vi "adjustAngle_03.vi"() -> ()   [LabVIEW 2011]
panel:
  out "dtArray":dbl[](array[numeric])
  out "t0":dbl
  in  "points to watch":i32
  in  "first":bool=TRUE
  in  "tArray":dbl[](array[numeric])
  out "tStart":dbl
  out "Measure":bool
  in  "Move to ref angle first":bool=TRUE
  in  "time done (s)":dbl
  in  "time to wait (s)":dbl=2.0
  out "Wait to set":bool
  in  "Ref Angle (deg)":dbl=30.0 format="%.1f"
  out "IO error":errorcluster
  in  "stop":bool
  out "Angle Indicator (deg)":dbl=20.6 caption="Angle (deg)" format="%.1f"
  in  "Angle (deg)":dbl format="%.1f"
  out "P (torr)":dbl=19.959999999999997 format="%.2f"
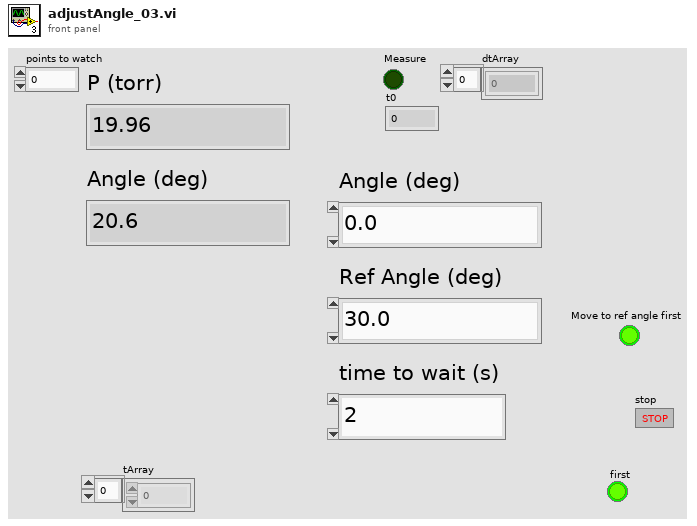
[diagram p1: front panel]
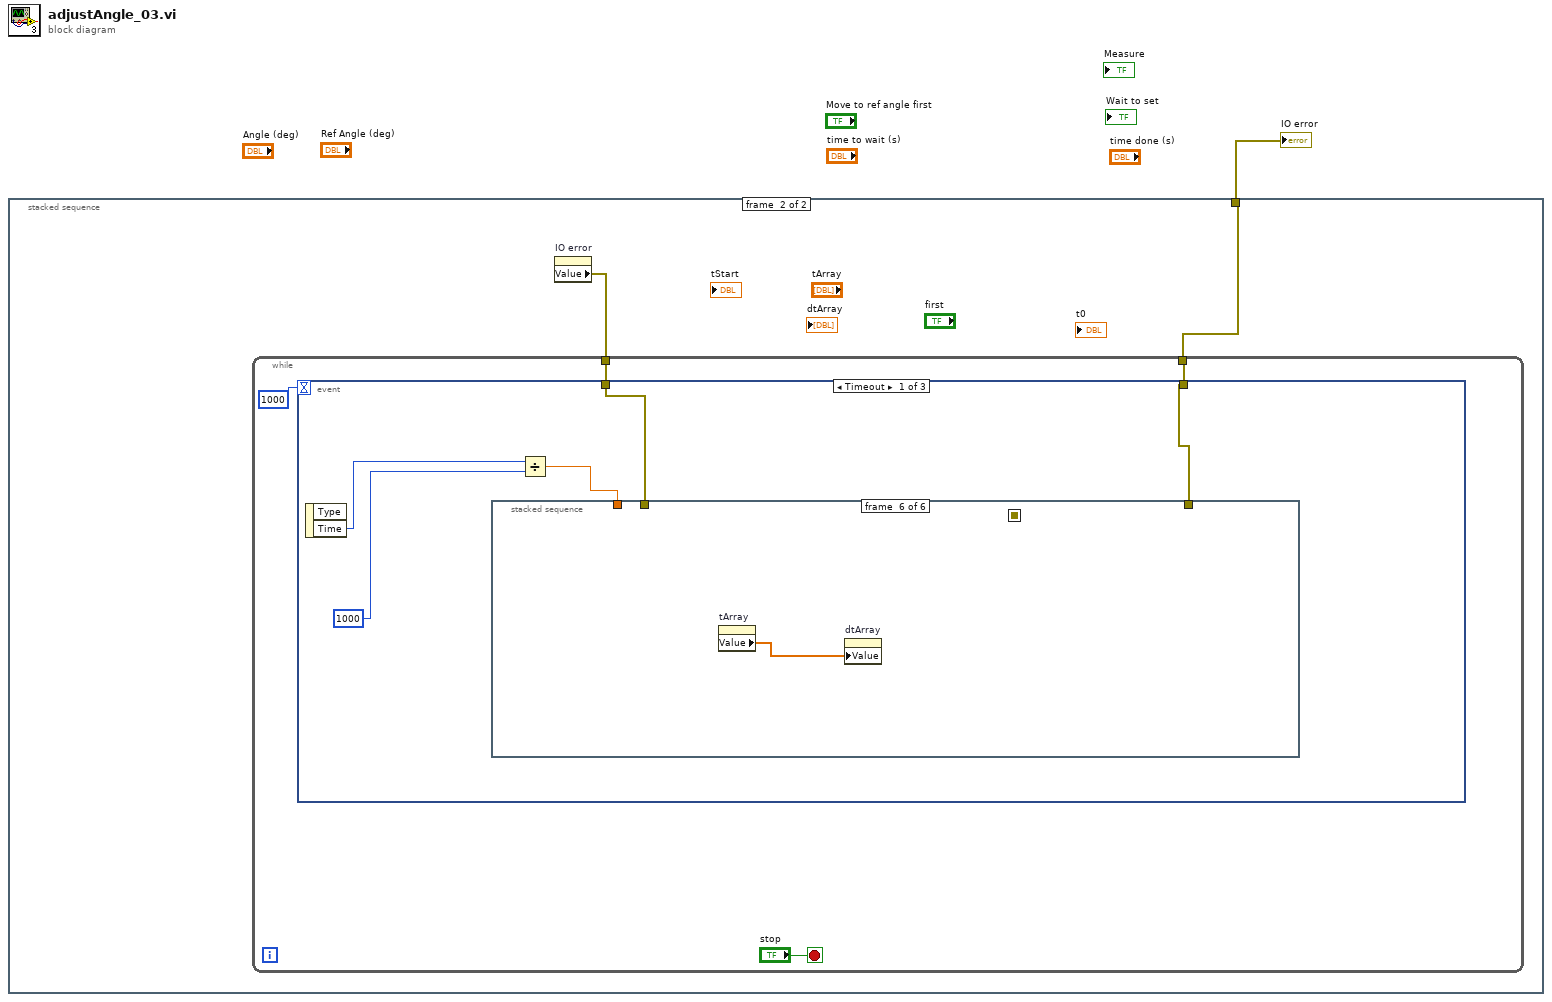
[diagram p0: block diagram]
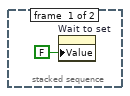
[diagram p2: hidden frame]
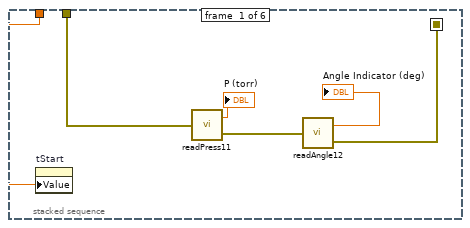
[diagram p3: hidden frame]
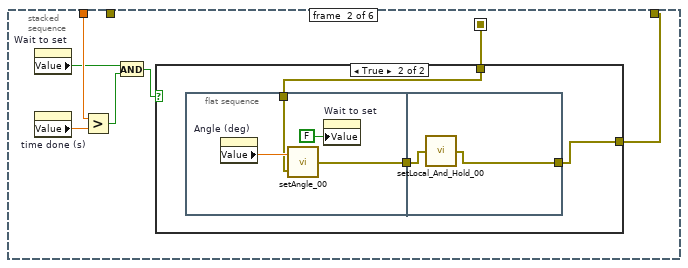
[diagram p4: hidden frame]
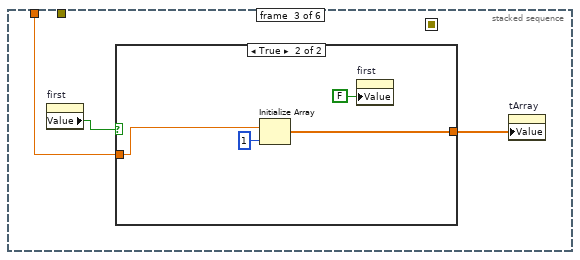
[diagram p6: hidden frame]
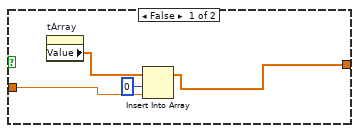
[diagram p7: hidden frame]
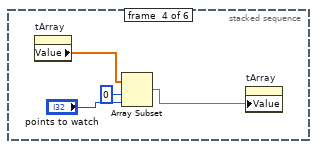
[diagram p8: hidden frame]
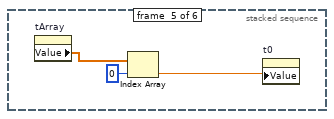
[diagram p9: hidden frame]
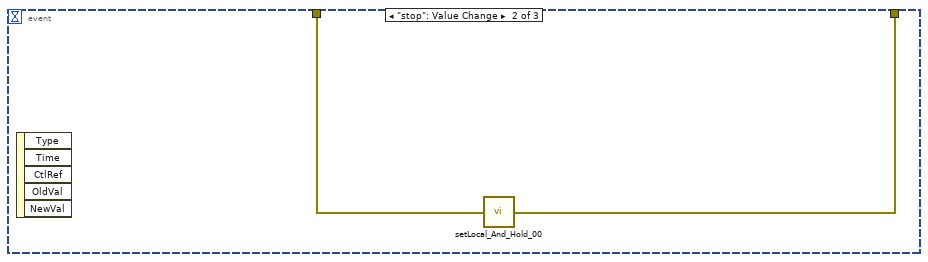
[diagram p10: hidden frame]
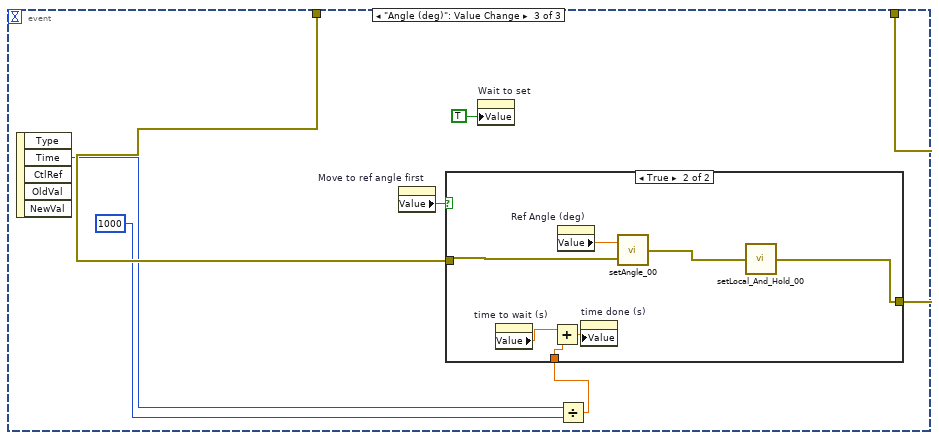
[diagram p11: hidden frame]
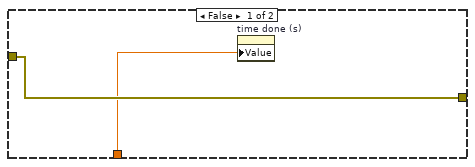
[diagram p12: hidden frame]
diagram:
  n1 = stacked-sequence {
    tunnel: [_ w3] -> w1
    frame #0 {
      n2 = property on="Wait to set" class="Bool (strict)"("Value"=FALSE ("Wait to set")) -> ()  [unwired: 2 in, 2 out]
    }
    frame #1 {
      n3 = property on="IO error" class="Clust (strict)"() -> ("Value"=w4:errorcluster)  [unwired: 2 in, 2 out]
      n4 = while {
        tunnel: w4 -> [w7]
        tunnel: [w6] -> w3
        stop <- "stop" stop-if-true
        n5 = event shown="[0] Timeout" {
          selector: _ -> [_ _ _]
          dyn-events: _ -> [_ _ _]
          timeout: 1000 -> [_ _ _]
          tunnel: w7 -> [w13 w57 w63]
          tunnel: [w12 w56 w64] -> w6
          event Timeout {
            n6 = event-data() -> ("Time"=w11:u32)  [unwired: 1 in, 1 out]
            n7 = Divide(x=w11, y=u32 1000) -> (x/y=w9:dbl)
            n8 = stacked-sequence {
              seq-local: [w15 _ _ _ _ _] -> [_ w20 _ _ _ _]
              tunnel: w13 -> [w19 _ _ _ _ _]
              tunnel: w9 -> [w14 w26 w39 _ _ _]
              tunnel: [_ w22 _ _ _ _] -> w12
              frame #0 {
                n9 = property on="tStart" class="DigNum (strict)"("Value"=w14) -> ()  [unwired: 2 in, 2 out]
                n10 = call "readPress11.vi"("error in"=w19) -> ("P"=→"P (torr)":dbl, "error out"=w16:errorcluster)
                n11 = call "readAngle12.vi"("error in"=w16) -> ("angle"=→"Angle Indicator (deg)":dbl, "error out"=w15:errorcluster)
              }
              frame #1 {
                n12 = property on="Wait to set" class="Bool (strict)"() -> ("Value"=w21:bool)  [unwired: 2 in, 2 out]
                n13 = property on="time done (s)" class="DigNum (strict)"() -> ("Value"=w25:dbl)  [unwired: 2 in, 2 out]
                n14 = Greater?(x=w26, y=w25) -> (0:w24:bool)
                n15 = And(x=w21, y=w24) -> (x .and. y?=w23:bool)
                n16 = case shown="True" w23 {
                  tunnel: [w27 w30] -> w22
                  tunnel: w20 -> [w27 w28]
                  frame False {
                  }
                  frame True {
                    n17 = flat-sequence {
                      tunnel: [w33] -> w29
                      tunnel: w28 -> [w31]
                      tunnel: [w35] -> w30
                      tunnel: w29 -> [w36]
                      frame #0 {
                        n18 = property on="Angle (deg)" class="DigNum (strict)"() -> ("Value"=w34:dbl)  [unwired: 2 in, 2 out]
                        n19 = call "setAngle_00.vi"("error in (no error)"=w31, "Angle (deg)"=w34) -> ("error out"=w33:errorcluster)
                        n20 = property on="Wait to set" class="Bool (strict)"("Value"=FALSE ("Wait to set")) -> ()  [unwired: 2 in, 2 out]
                      }
                      frame #1 {
                        n21 = call "setLocal_And_Hold_00.vi"("error in (no error)"=w36) -> ("error out"=w35:errorcluster)
                      }
                    }
                  }
                }
              }
              frame #2 {
                n22 = property on="first" class="Bool (strict)"() -> ("Value"=w38:bool)  [unwired: 2 in, 2 out]
                n23 = case shown="True" w38 {
                  tunnel: w39 -> [w43 w47]
                  tunnel: [w40 w45] -> w37
                  frame False {
                    n24 = property on="tArray" class="Arr (strict)"() -> ("Value"=w42:dbl[])  [unwired: 2 in, 2 out]
                    n25 = Insert Into Array(array=w42, index=0, new element=w43) -> (w40:dbl[])
                  }
                  frame True {
                    n26 = Initialize Array(w47, 1 ("dimension size")) -> (w45:dbl[])
                    n27 = property on="first" class="Bool (strict)"("Value"=FALSE ("first")) -> ()  [unwired: 2 in, 2 out]
                  }
                }
                n28 = property on="tArray" class="Arr (strict)"("Value"=w37) -> ()  [unwired: 2 in, 2 out]
              }
              frame #3 {
                n29 = property on="tArray" class="Arr (strict)"() -> ("Value"=w49:dbl[])  [unwired: 2 in, 2 out]
                n30 = Array Subset(array=w49, index=0, length="points to watch") -> (w48:dbl[])
                n31 = property on="tArray" class="Arr (strict)"("Value"=w48) -> ()  [unwired: 2 in, 2 out]
              }
              frame #4 {
                n32 = property on="tArray" class="Arr (strict)"() -> ("Value"=w54:dbl[])  [unwired: 2 in, 2 out]
                n33 = Index Array(array=w54, index=0) -> (element=w52:dbl)
                n34 = property on="t0" class="DigNum (strict)"("Value"=w52) -> ()  [unwired: 2 in, 2 out]
              }
              frame #5 {
                n35 = property on="tArray" class="Arr (strict)"() -> ("Value"=w55:dbl[])  [unwired: 2 in, 2 out]
                n36 = property on="dtArray" class="Arr (strict)"("Value"=w55) -> ()  [unwired: 2 in, 2 out]
              }
            }
          }
          event "stop": Value Change {
            n37 = event-data() -> ()  [unwired: 1 in, 5 out]
            n38 = call "setLocal_And_Hold_00.vi"("error in (no error)"=w57) -> ("error out"=w56:errorcluster)
          }
          event "Angle (deg)": Value Change {
            n39 = event-data() -> ("Time"=w62:u32)  [unwired: 1 in, 4 out]
            n40 = property on="Move to ref angle first" class="Bool (strict)"() -> ("Value"=w59:bool)  [unwired: 2 in, 2 out]
            n41 = property on="Wait to set" class="Bool (strict)"("Value"=TRUE ("Wait to set")) -> ()  [unwired: 2 in, 2 out]
            n42 = Divide(x=w62, y=u32 1000) -> (x/y=w60:dbl)
            n43 = case shown="True" w59 {
              tunnel: w63 -> [w66 w72]
              tunnel: [w66 w67] -> w64
              tunnel: w60 -> [w65 w69]
              frame False {
                n44 = property on="time done (s)" class="DigNum (strict)"("Value"=w65) -> ()  [unwired: 2 in, 2 out]
              }
              frame True {
                n45 = property on="time to wait (s)" class="DigNum (strict)"() -> ("Value"=w70:dbl)  [unwired: 2 in, 2 out]
                n46 = Add(x=w70, y=w69) -> (x+y=w71:dbl)
                n47 = property on="Ref Angle (deg)" class="DigNum (strict)"() -> ("Value"=w73:dbl)  [unwired: 2 in, 2 out]
                n48 = property on="time done (s)" class="DigNum (strict)"("Value"=w71) -> ()  [unwired: 2 in, 2 out]
                n49 = call "setAngle_00.vi"("error in (no error)"=w72, "Angle (deg)"=w73) -> ("error out"=w68:errorcluster)
                n50 = call "setLocal_And_Hold_00.vi"("error in (no error)"=w68) -> ("error out"=w67:errorcluster)
              }
            }
          }
        }
      }
    }
  }
  "IO error" <- w1
